vi "GetRightClickMenu.vi"(0 "reference":refnum<class "Graph.lvclass">, 5 "error in (no error)":errorcluster) -> (14 "reference out":refnum<class "Graph.lvclass">, 15 "Array":string[](array[string]), 16 "Found":bool, 19 "error out":errorcluster)   [LabVIEW 2014, in "Graph.lvclass"]
doc: "GetRightClickMenu"
uses:
  <resource>/Framework/Providers/Open_GDS/UML/Graph_class/Graph.lvclass
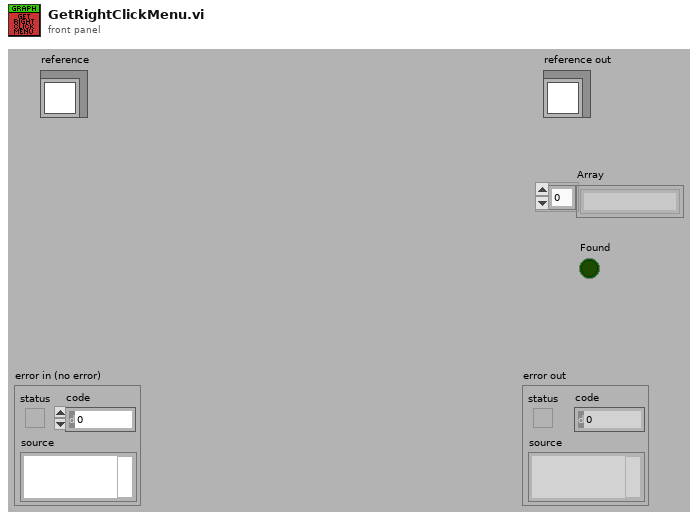
[diagram p1: front panel]
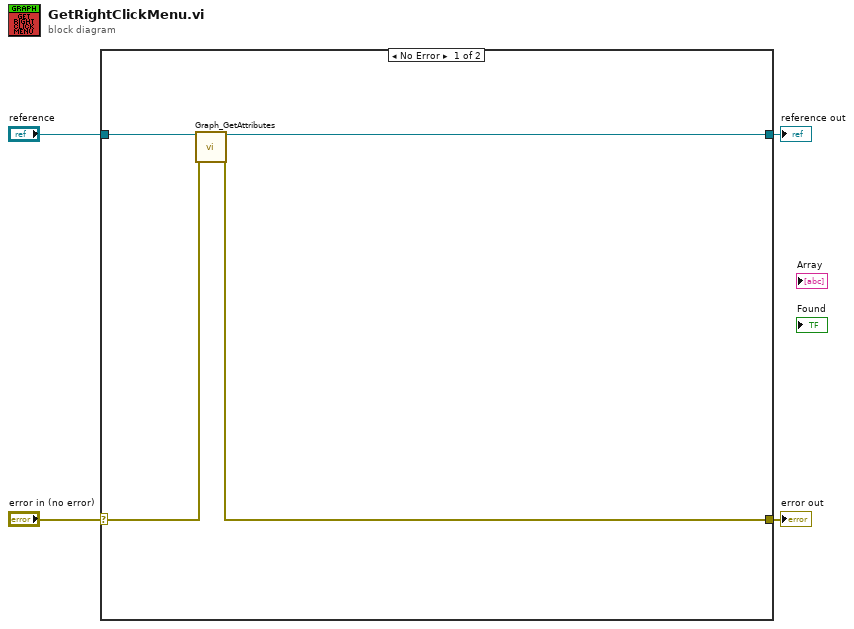
[diagram p0: block diagram]
diagram:
  n1 = case shown="No Error" "error in (no error)" {
    selector: "error in (no error)" -> [w5 w9]
    tunnel: "reference" -> [w8 w10]
    tunnel: [w7 w9] -> w3
    tunnel: [w6 w10] -> w2
    frame No Error {
      n2 = call <resource>:"Graph_GetAttributes.vi"("reference in"=w8, "error in (no error)"=w5) -> ("reference out"=w6:refnum<class "Graph.lvclass">, "error out"=w7:errorcluster)  [unwired: 16 out]
    }
    frame Error {
    }
  }
  "reference out" <- w2
  "error out" <- w3
